vi "Path2Str(2last).vi"(3 "Sequence":path) -> (1 "String":string)   [LabVIEW 2019, in "Tools.lvlib"]
uses:
  Tools.lvlib
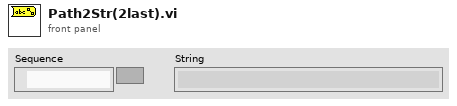
[diagram p1: front panel]
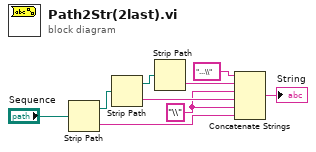
[diagram p0: block diagram]
diagram:
  w1 = "\\" ("string")
  n1 = Strip Path(path="Sequence") -> (stripped path=w8:path, name=w6:string)
  n2 = Strip Path(path=w8) -> (stripped path=w3:path, name=w7:string)
  n3 = Strip Path(path=w3) -> (name=w2:string)  [unwired: 1 out]
  n4 = Concatenate Strings("...\\" ("string"), w2, w1, w7, w1, w6) -> (→"String":string)
